vi "Save Settings to File.vi"(8 "error in (no error)":errorcluster, 11 "Application in":refnum<class "Application.lvclass">) -> (0 "error out":errorcluster, 3 "Application out":refnum<class "Application.lvclass">)   [LabVIEW 2017, in "Application.lvlib" / "Application.lvclass"]
doc: "Saves the current settings of an Application to file using a persistance object."
uses:
  Application.lvclass
  C:/Program Files (x86)/National Instruments/LabVIEW 2017/vi.lib/TSS/ACRObat Test Framework/Classes/Base Objects/Base Class/Base Class/Base Class.lvclass
  <vilib>/TSS/ACRObat Test Framework/Utilities/Data Persistance/Settings Data/Settings Data.lvclass
  Application.lvclass/Application.ctl
  Settings/App Settings.lvclass
  <vilib>/TSS/ACRObat Test Framework/Classes/Base Objects/Base Class/Base Class/Base Class.lvclass
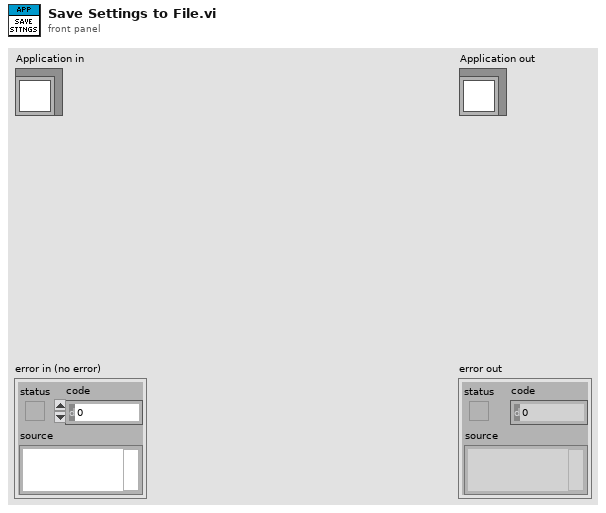
[diagram p1: front panel]
types:
  T1 = typedef "Application.lvlib/App Settings.lvclass/Class Settings -- Cluster.ctl" = cluster{"DataLogging Enabled":bool, "AutoStart":bool, "AutoClear":bool, "Cycle Timeout":u32, "Wait Before Clear":u32, "Machine ID":string, "Test Type":string, "Product Name":string, "Meta Tags":string[], "Meta Values":string[], "Viewer Settings":cluster{"DataViewer Headers":string[], "Pass Fail Settings":T2}}
  T2 = typedef "Data Viewer.lvlib/Data Viewer Settings.lvclass/Pass Fail Criteria -- Cluster.ctl" = cluster{"Header":string, "Criteria":string}
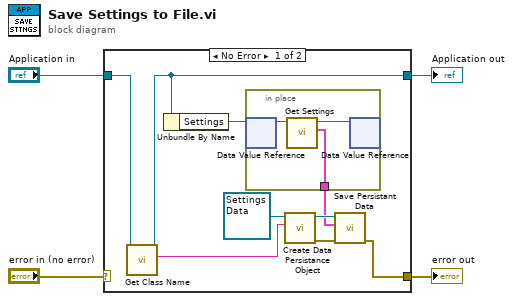
[diagram p0: block diagram]
diagram:
  n1 = case shown="No Error" "error in (no error)" {
    selector: "error in (no error)" -> [_ w18]
    tunnel: [w5 w18] -> w3
    tunnel: [w12 w17] -> w1
    tunnel: "Application in" -> [w13 w17]
    frame No Error {
      n2 = call <vilib>:"Get Class Name.vi"("Base Class in"=w13) -> ("Qualified Name"=w11:string, "Base Class out"=w12:refnum<class "Application.lvclass">)  [unwired: 8 in, 1 out]
      n3 = Unbundle By Name(w12) -> ("Settings"=w9:refnum<data-value>)
      n4 = in-place {
        in-place-border: [w14] -> w8
        n5 = in-place-dvr #1(w9) -> (w16:refnum<class "App Settings.lvclass">)  [unwired: 1 out]
        n6 = call-dynamic "Get Settings.vi"("App Settings in"=w16) -> ("Settings"=w14:T1, "App Settings out"=w15:refnum<class "App Settings.lvclass">)  [unwired: 8 in, 1 out]
        n7 = in-place-dvr #1(w15) -> ()  [unwired: 2 out]
      }
      n8 = call-dynamic "Create Data Persistance Object.vi"("Object Name"=w11, "Settings Data in"=refnum<class "Settings Data.lvclass"> refnum) -> ("error out"=w6:errorcluster, "Settings Data out"=w10:refnum<class "Settings Data.lvclass">)  [unwired: 8 in]
      n9 = call-dynamic "Save Persistant Data.vi"("error in (no error)"=w6, "Data"=w8, "Data Persistance in"=w10) -> ("error out"=w5:errorcluster)  [unwired: 7 in, 1 out]
    }
    frame Error {
    }
  }
  "error out" <- w3
  "Application out" <- w1
